vi "TSCAN_GetCANDBInfo.vi"(8 "ADatabaseld":u32=1, 10 "Path":path) -> (0 "ID":i32[](array[numeric]) format="%x", 1 "SignalName":string[][](array[string]), 2 "Message":string[](array[string]), 3 "Path output":path, 4 "Message&ID":string[](array[string]), 5 "ALLName":string[](array[string]))   [LabVIEW 2014]
uses:
  <vilib>/Utility/importsl/GetValueByPointer/GetValueByPointer.xnode
  <vilib>/Utility/importsl/GetValueByPointer/datatype.ctl
panel:
  in  "QueryType":i32(ring) items=["DT_STR_Network_Name", "DT_STR_DBC_FileName", "DT_INT_Protocol_Type", "DT_INT_3", "DT_INT_4", "DT_INT_5", "DT_INT_6", "DT_INT_7", "DT_INT_8", "DT_INT_9", "DT_INT_Signal_List_Count", "DT_INT_CAN_Message_List_Count", "DT_INT_CANFD_Message_List_Count", "DT_INT_CANJ1939_Message_List_Count", "DT_INT_Node_List_Count", "DT_INT_EnvVar_List_Count", "DT_INT_ValTab_List_Count", "DT_INT_17", "DT_INT_18", "DT_INT_19", "DT_INT_Signal_List_Message_ID", "DT_INT_Signal_List_Value_Type", "DT_INT_Signal_List_Is_Motorola", "DT_INT_Signal_List_ValTab_Index", "DT_INT_Signal_List_Mux_Type", "DT_INT_Signal_List_Mux_Value", "DT_INT_Signal_List_Layout_Start", "DT_INT_Signal_List_Length", "DT_DBL_Signal_List_Factor", "DT_DBL_Signal_List_Offset", "DT_DBL_Signal_List_InitValue", "DT_DBL_Signal_List_Min", "DT_DBL_Signal_List_Max", "DT_STR_Signal_List_Name", "DT_STR_Signal_List_Unit", "DT_STR_Signal_List_Comment", "DT_INT_Signal_List_Message_Index", "DT_INT_Signal_List_Message_Type", "DT_STR_Signal_List_Struct", "DT_INT_39", "DT_INT_CAN_Message_List_Type", "DT_INT_CAN_Message_List_DLC", "DT_INT_CAN_Message_List_ID", "DT_INT_CAN_Message_List_CycleTime", "DT_STR_CAN_Message_List_Name", "DT_STR_CAN_Message_List_Comment", "DT_INT_CAN_Message_List_TX_Node_Index", "DT_INT_CAN_Message_List_Owned_Signal_List_Count", "DT_INT_CAN_Message_List_Owned_Signal_List_Signal_Index", "DT_STR_CAN_Message_List_Struct", "DT_INT_50", "DT_INT_51", "DT_INT_52", "DT_INT_53", "DT_INT_54", "DT_INT_55", "DT_INT_56", "DT_INT_57", "DT_INT_58", "DT_INT_59", "DT_INT_CANFD_Message_List_Type", "DT_INT_CANFD_Message_List_DLC", "DT_INT_CANFD_Message_List_ID", "DT_INT_CANFD_Message_List_CycleTime", "DT_STR_CANFD_Message_List_Name", "DT_STR_CANFD_Message_List_Comment", "DT_INT_CANFD_Message_List_TX_Node_Index", "DT_INT_CANFD_Message_List_Owned_Signal_List_Count", "DT_INT_CANFD_Message_List_Owned_Signal_List_Signal_Index", "DT_INT_CANFD_Message_List_BRS", "DT_STR_CANFD_Message_List_Struct", "DT_INT_71", "DT_INT_72", "DT_INT_73", "DT_INT_74", "DT_INT_75", "DT_INT_76", "DT_INT_77", "DT_INT_78", "DT_INT_79", "DT_INT_J1939_Message_List_Type", "DT_INT_J1939_Message_List_DLC", "DT_INT_J1939_Message_List_ID", "DT_INT_J1939_Message_List_CycleTime", "DT_STR_J1939_Message_List_Name", "DT_STR_J1939_Message_List_Comment", "DT_INT_J1939_Message_List_TX_Node_Index", "DT_INT_J1939_Message_List_Owned_Signal_List_Count", "DT_INT_J1939_Message_List_Owned_Signal_List_Signal_Index", "DT_STR_J1939_Message_List_Struct", "DT_INT_90", "DT_INT_91", "DT_INT_92", "DT_INT_93", "DT_INT_94", "DT_INT_95", "DT_INT_96", "DT_INT_97", "DT_INT_98", "DT_INT_99", "DT_INT_Node_List_Address", "DT_STR_Node_List_Name", "DT_STR_Node_List_Comment", "DT_INT_Node_List_TX_CAN_Message_List_Count", "DT_INT_Node_List_TX_CAN_Message_List_Message_Index", "DT_INT_Node_List_RX_CAN_Message_List_Count", "DT_INT_Node_List_RX_CAN_Message_List_Message_Index", "DT_INT_Node_List_TX_FD_Message_List_Count", "DT_INT_Node_List_TX_FD_Message_List_Message_Index", "DT_INT_Node_List_RX_FD_Message_List_Count", "DT_INT_Node_List_RX_FD_Message_List_Message_Index", "DT_INT_Node_List_TX_J1939_Message_List_Count", "DT_INT_Node_List_TX_J1939_Message_List_Message_Index", "DT_INT_Node_List_RX_J1939_Message_List_Count", "DT_INT_Node_List_RX_J1939_Message_List_Message_Index", "DT_INT_Node_List_TX_Signal_List_Count", "DT_INT_Node_List_TX_Signal_List_Signal_Index", "DT_INT_Node_List_RX_Signal_List_Count", "DT_INT_Node_List_RX_Signal_List_Signal_Index", "DT_STR_Node_List_Struct", "DT_INT_120", "DT_INT_121", "DT_INT_122", "DT_INT_123", "DT_INT_124", "DT_INT_125", "DT_INT_126", "DT_INT_127", "DT_INT_128", "DT_INT_129", "DT_INT_EnvVar_List_Value_Type", "DT_DBL_EnvVar_List_MIN", "DT_DBL_EnvVar_List_MAX", "DT_DBL_EnvVar_List_Init_Value", "DT_STR_EnvVar_List_Name", "DT_STR_EnvVar_List_Unit", "DT_STR_EnvVar_List_Comment", "DT_STR_EnvVar_List_Struct", "DT_INT_138", "DT_INT_139", "DT_INT_ValTab_List_Item_List_Count", "DT_INT_ValTab_List_Item_List_Name", "DT_DBL_ValTab_List_Item_List_Value", "DT_STR_ValTab_List_Struct"]
  out "错误输出":errorcluster
  out "tsdb_load_can_db 2":i32
  out "tsdb_load_can_db":i32
  # "Same Mssage in the same row"
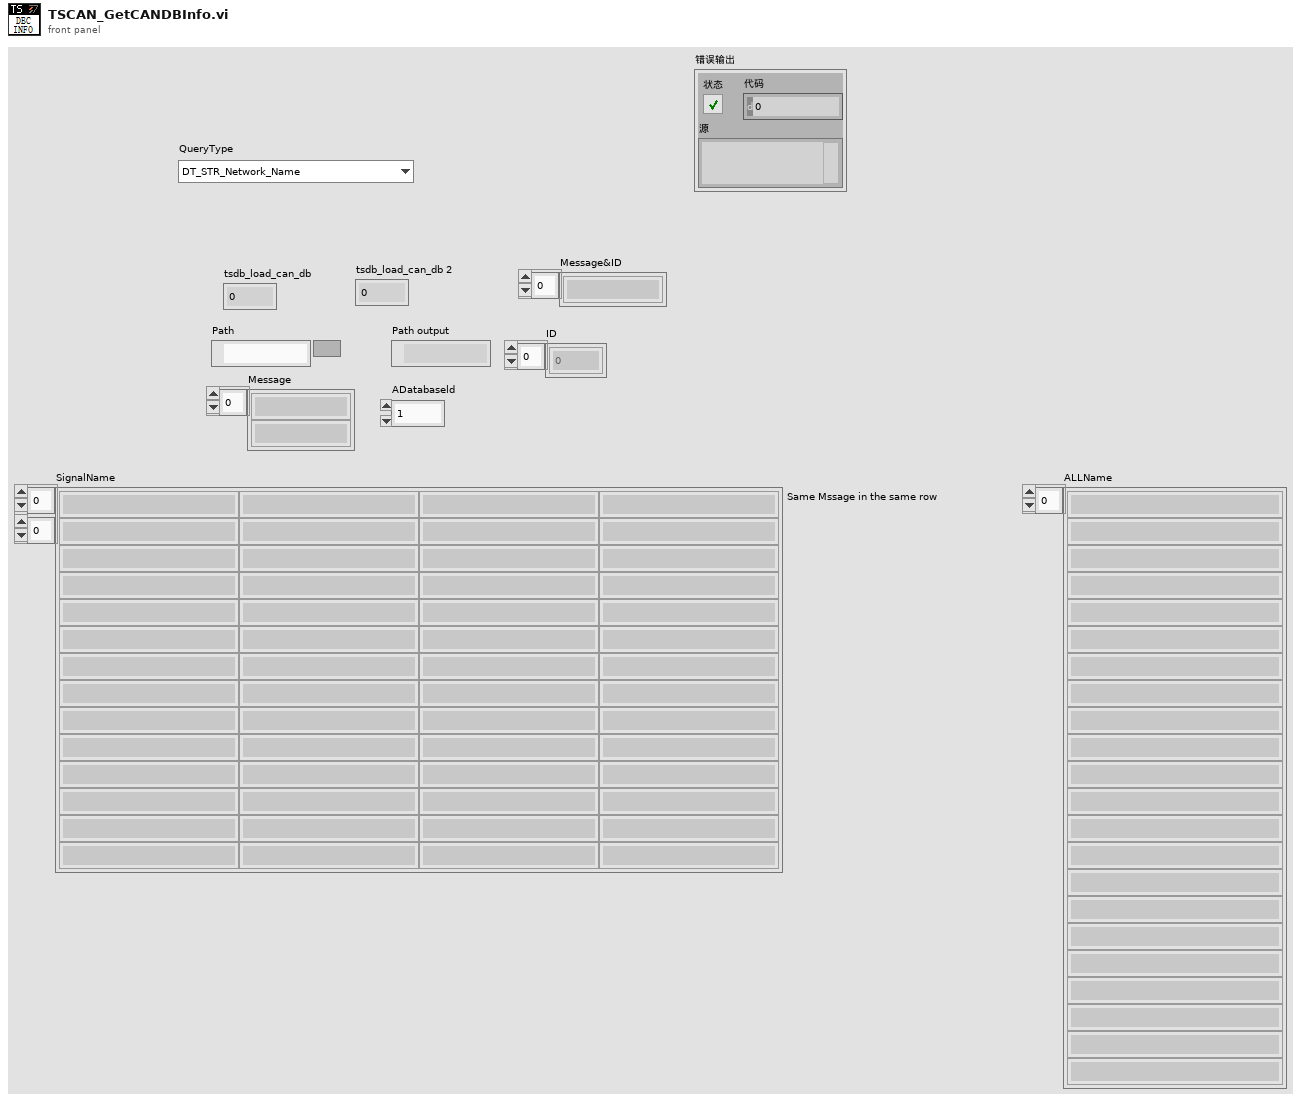
[diagram p1: front panel]
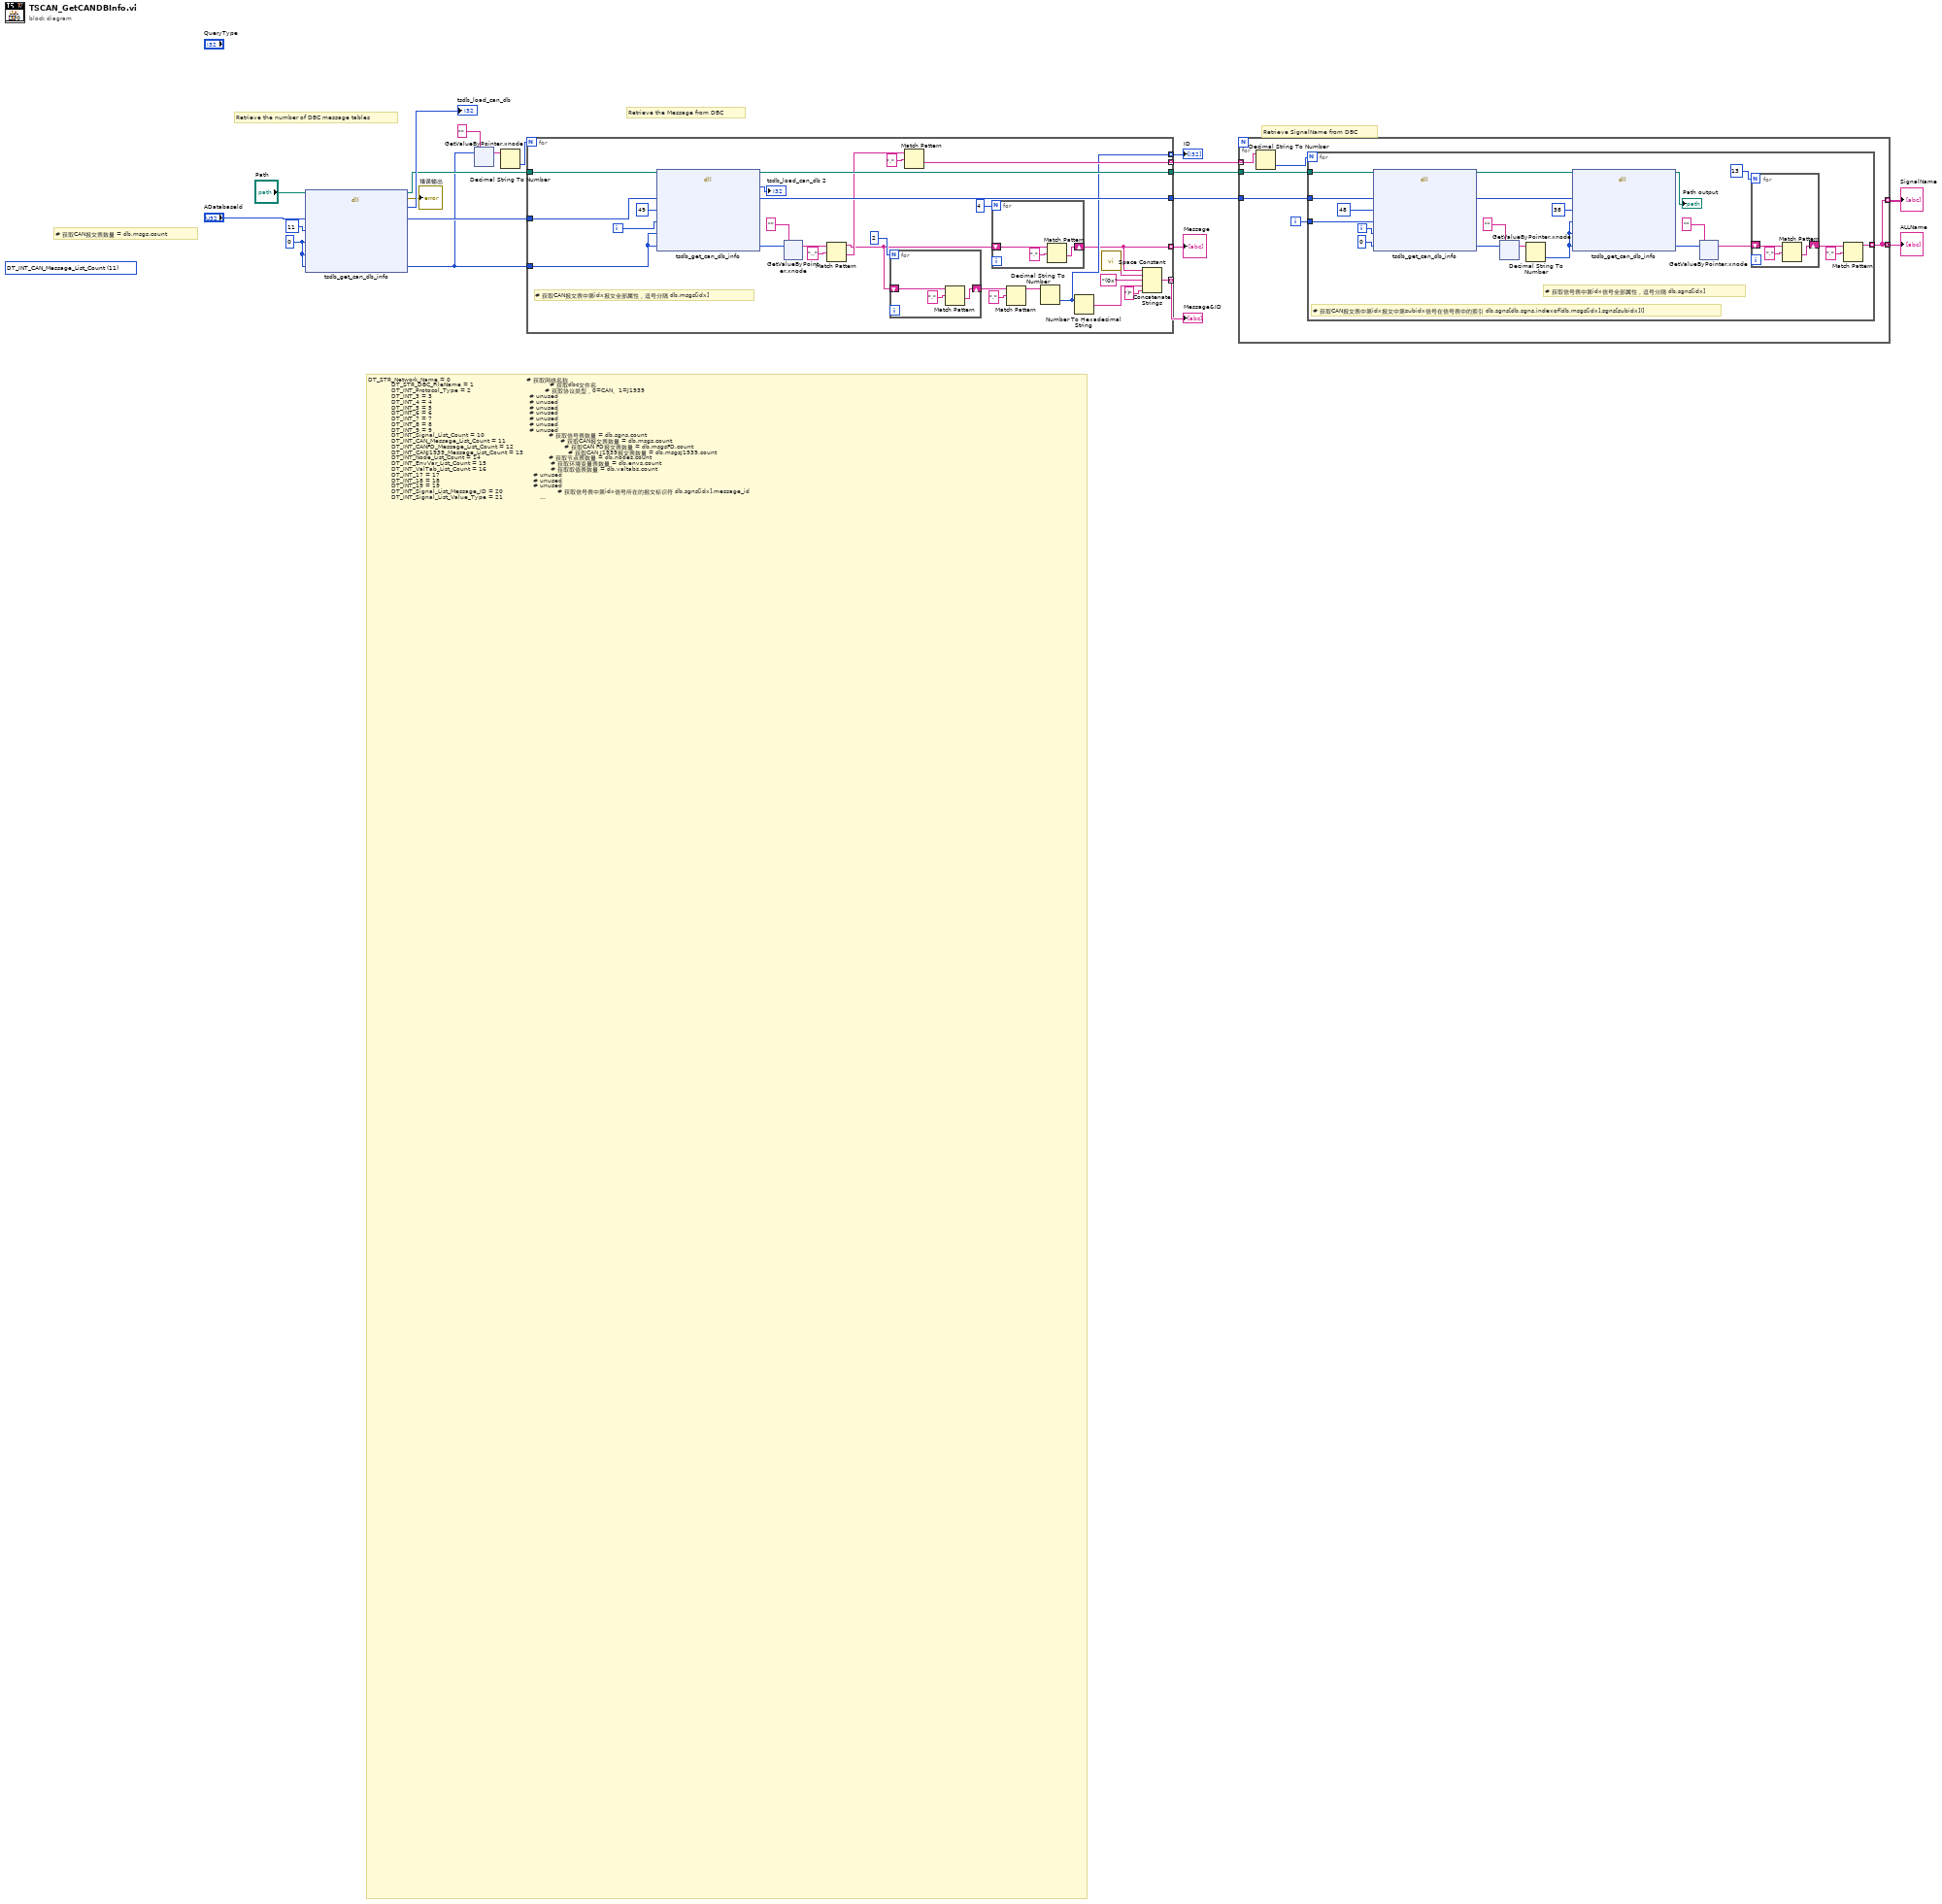
[diagram p0: block diagram]
diagram:
  (unwired) 11 items=["DT_STR_Network_Name", "DT_STR_DBC_FileName", "DT_INT_Protocol_Type", "DT_INT_3", "DT_INT_4", "DT_INT_5", "DT_INT_6", "DT_INT_7", "DT_INT_8", "DT_INT_9", "DT_INT_Signal_List_Count", "DT_INT_CAN_Message_List_Count", "DT_INT_CANFD_Message_List_Count", "DT_INT_CANJ1939_Message_List_Count", "DT_INT_Node_List_Count", "DT_INT_EnvVar_List_Count", "DT_INT_ValTab_List_Count", "DT_INT_17", "DT_INT_18", "DT_INT_19", "DT_INT_Signal_List_Message_ID", "DT_INT_Signal_List_Value_Type", "DT_INT_Signal_List_Is_Motorola", "DT_INT_Signal_List_ValTab_Index", "DT_INT_Signal_List_Mux_Type", "DT_INT_Signal_List_Mux_Value", "DT_INT_Signal_List_Layout_Start", "DT_INT_Signal_List_Length", "DT_DBL_Signal_List_Factor", "DT_DBL_Signal_List_Offset", "DT_DBL_Signal_List_InitValue", "DT_DBL_Signal_List_Min", "DT_DBL_Signal_List_Max", "DT_STR_Signal_List_Name", "DT_STR_Signal_List_Unit", "DT_STR_Signal_List_Comment", "DT_INT_Signal_List_Message_Index", "DT_INT_Signal_List_Message_Type", "DT_STR_Signal_List_Struct", "DT_INT_39", "DT_INT_CAN_Message_List_Type", "DT_INT_CAN_Message_List_DLC", "DT_INT_CAN_Message_List_ID", "DT_INT_CAN_Message_List_CycleTime", "DT_STR_CAN_Message_List_Name", "DT_STR_CAN_Message_List_Comment", "DT_INT_CAN_Message_List_TX_Node_Index", "DT_INT_CAN_Message_List_Owned_Signal_List_Count", "DT_INT_CAN_Message_List_Owned_Signal_List_Signal_Index", "DT_STR_CAN_Message_List_Struct", "DT_INT_50", "DT_INT_51", "DT_INT_52", "DT_INT_53", "DT_INT_54", "DT_INT_55", "DT_INT_56", "DT_INT_57", "DT_INT_58", "DT_INT_59", "DT_INT_CANFD_Message_List_Type", "DT_INT_CANFD_Message_List_DLC", "DT_INT_CANFD_Message_List_ID", "DT_INT_CANFD_Message_List_CycleTime", "DT_STR_CANFD_Message_List_Name", "DT_STR_CANFD_Message_List_Comment", "DT_INT_CANFD_Message_List_TX_Node_Index", "DT_INT_CANFD_Message_List_Owned_Signal_List_Count", "DT_INT_CANFD_Message_List_Owned_Signal_List_Signal_Index", "DT_INT_CANFD_Message_List_BRS", "DT_STR_CANFD_Message_List_Struct", "DT_INT_71", "DT_INT_72", "DT_INT_73", "DT_INT_74", "DT_INT_75", "DT_INT_76", "DT_INT_77", "DT_INT_78", "DT_INT_79", "DT_INT_J1939_Message_List_Type", "DT_INT_J1939_Message_List_DLC", "DT_INT_J1939_Message_List_ID", "DT_INT_J1939_Message_List_CycleTime", "DT_STR_J1939_Message_List_Name", "DT_STR_J1939_Message_List_Comment", "DT_INT_J1939_Message_List_TX_Node_Index", "DT_INT_J1939_Message_List_Owned_Signal_List_Count", "DT_INT_J1939_Message_List_Owned_Signal_List_Signal_Index", "DT_STR_J1939_Message_List_Struct", "DT_INT_90", "DT_INT_91", "DT_INT_92", "DT_INT_93", "DT_INT_94", "DT_INT_95", "DT_INT_96", "DT_INT_97", "DT_INT_98", "DT_INT_99", "DT_INT_Node_List_Address", "DT_STR_Node_List_Name", "DT_STR_Node_List_Comment", "DT_INT_Node_List_TX_CAN_Message_List_Count", "DT_INT_Node_List_TX_CAN_Message_List_Message_Index", "DT_INT_Node_List_RX_CAN_Message_List_Count", "DT_INT_Node_List_RX_CAN_Message_List_Message_Index", "DT_INT_Node_List_TX_FD_Message_List_Count", "DT_INT_Node_List_TX_FD_Message_List_Message_Index", "DT_INT_Node_List_RX_FD_Message_List_Count", "DT_INT_Node_List_RX_FD_Message_List_Message_Index", "DT_INT_Node_List_TX_J1939_Message_List_Count", "DT_INT_Node_List_TX_J1939_Message_List_Message_Index", "DT_INT_Node_List_RX_J1939_Message_List_Count", "DT_INT_Node_List_RX_J1939_Message_List_Message_Index", "DT_INT_Node_List_TX_Signal_List_Count", "DT_INT_Node_List_TX_Signal_List_Signal_Index", "DT_INT_Node_List_RX_Signal_List_Count", "DT_INT_Node_List_RX_Signal_List_Signal_Index", "DT_STR_Node_List_Struct", "DT_INT_120", "DT_INT_121", "DT_INT_122", "DT_INT_123", "DT_INT_124", "DT_INT_125", "DT_INT_126", "DT_INT_127", "DT_INT_128", "DT_INT_129", "DT_INT_EnvVar_List_Value_Type", "DT_DBL_EnvVar_List_MIN", "DT_DBL_EnvVar_List_MAX", "DT_DBL_EnvVar_List_Init_Value", "DT_STR_EnvVar_List_Name", "DT_STR_EnvVar_List_Unit", "DT_STR_EnvVar_List_Comment", "DT_STR_EnvVar_List_Struct", "DT_INT_138", "DT_INT_139", "DT_INT_ValTab_List_Item_List_Count", "DT_INT_ValTab_List_Item_List_Name", "DT_DBL_ValTab_List_Item_List_Value", "DT_STR_ValTab_List_Struct"] ("QueryType")
  w8 = u32 0 ("AIndex")
  # "# 获取CAN报文表数量 = db.msgs.count"
  # "DT_STR_Network_Name = 0                                       # 获取网络名称\n            DT_STR_DBC_FileName = 1                                       # 获取dbc文件名\n            DT_INT_Protocol_Type = 2                                      # 获取协议类型，0=CAN、1=J1939\n            DT_INT_3 = 3                                                  # unused\n            DT_INT_4 = 4                                                  # unused\n            DT_INT_5 = 5                                                  # unused\n            DT_INT_6 = 6                                                  # unused\n            DT_INT_7 = 7                                                  # unused\n            DT_INT_8 = 8                                                  # unused\n            DT_INT_9 = 9                                                  # unused\n            DT_INT_Signal_List_Count = 10                                 # 获取信号表数量 = db.sgns.count\n            DT_INT_CAN_Message_List_Count = 11                            # 获取CAN报文表数量 = db.msgs.count\n            DT_INT_CANFD_Message_List_Count = 12                          # 获取CAN FD报文表数量 = db.msgsFD.count\n            DT_INT_CANJ1939_Message_List_Count = 13                       # 获取CAN J1939报文表数量 = db.msgsJ1939.count\n            DT_INT_Node_List_Count = 14                                   # 获取节点表数量 = db.nodes.count\n            DT_INT_EnvVar_List_Count = 15                                 # 获取环境变量表数量 = db.envs.count\n            DT_INT_ValTab_List_Count = 16                                 # 获取取值表数量 = db.valtabs.count\n            DT_INT_17 = 17                                                # unused\n            DT_INT_18 = 18                                                # unused\n            DT_INT_19 = 19                                                # unused\n            DT_INT_Signal_List_Message_ID = 20                            # 获取信号表中第idx信号所在的报文标识符 db.sgns[idx].message_id\n            DT_INT_Signal_List_Value_Type = 21                            # 获取信号表中第idx信号值类型 0-无符号整型 1-有符号整型 2-32位浮点 3-64位浮点\n            DT_INT_Signal_List_Is_Motorola = 22                           # 获取信号表中第idx信号是否是Motorola格式，0-Intel格式、1-Motorola格式\n            DT_INT_Signal_List_ValTab_Index = 23                          # 获取信号表中第idx信号所带的取值表在取值表列表中的索引\n            DT_INT_Signal_List_Mux_Type = 24                              # 获取信号表中第idx信号Mux类型，0-普通信号 1-multiplexor 2-multiplexed信号\n            DT_INT_Signal_List_Mux_Value = 25                             # 获取信号表中第idx信号作为multiplexor的值\n            DT_INT_Signal_List_Layout_Start = 26                          # 获取信号表中第idx信号在报文中的起始位\n            DT_INT_Signal_List_Length = 27                                # 获取信号表中第idx信号的信号长度\n            DT_DBL_Signal_List_Factor = 28                                # 获取信号表中第idx信号放大因子\n            DT_DBL_Signal_List_Offset = 29                                # 获取信号表中第idx信号偏移量\n            DT_DBL_Signal_List_InitValue = 30                             # 获取信号表中第idx信号初始值\n            DT_DBL_Signal_List_Min = 31                                   # 获取信号表中第idx信号最小值\n            DT_DBL_Signal_List_Max = 32                                   # 获取信号表中第idx信号最大值\n            DT_STR_Signal_List_Name = 33                                  # 获取信号表中第idx信号名称\n            DT_STR_Signal_List_Unit = 34                                  # 获取信号表中第idx信号单位\n            DT_STR_Signal_List_Comment = 35                               # 获取信号表中第idx信号注释\n            DT_INT_Signal_List_Message_Index = 36                         # 获取信号表中第idx信号所在的报文在报文表中的索引 db.msgs[db.sgns[idx].message_idx]\n            DT_INT_Signal_List_Message_Type = 37                          # 获取信号表中第idx信号所在的报文的类型，0=CAN 1=CANFD 2=J1939\n            DT_STR_Signal_List_Struct = 38                                # 获取信号表中第idx信号全部属性，逗号分隔 db.sgns[idx]\n            DT_INT_39 = 39                                                # unused\n            DT_INT_CAN_Message_List_Type = 40                             # 获取CAN报文表中第idx报文类型，cftStdCAN = 0 cftExtCAN = 1 cftJ1939 = 2 cftStdCANFD = 3 cftExtCANFD = 4\n            DT_INT_CAN_Message_List_DLC = 41                              # 获取CAN报文表中第idx报文数据长度\n            DT_INT_CAN_Message_List_ID = 42                               # 获取CAN报文表中第idx报文标识符\n            DT_INT_CAN_Message_List_CycleTime = 43                        # 获取CAN报文表中第idx报文周期\n            DT_STR_CAN_Message_List_Name = 44                             # 获取CAN报文表中第idx报文名称\n            DT_STR_CAN_Message_List_Comment = 45                          # 获取CAN报文表中第idx报文注释\n            DT_INT_CAN_Message_List_TX_Node_Index = 46                    # 获取CAN报文表中第idx报文对应的发送节点的索引\n            DT_INT_CAN_Message_List_Owned_Signal_List_Count = 47          # 获取CAN报文表中第idx报文拥有的信号数量 db.msgs[idx].sgns.count\n            DT_INT_CAN_Message_List_Owned_Signal_List_Signal_Index = 48   # 获取CAN报文表中第idx报文中第subidx信号在信号表中的索引 db.sgns[db.sgns.indexof(db.msgs[idx].sgns[subidx])]\n            DT_STR_CAN_Message_List_Struct = 49                           # 获取CAN报文表中第idx报文全部属性，逗号分隔 db.msgs[idx]\n            DT_INT_50 = 50                                                # unused\n            DT_INT_51 = 51                                                # unused\n            DT_INT_52 = 52                                                # unused\n            DT_INT_53 = 53                                                # unused\n            DT_INT_54 = 54                                                # unused\n            DT_INT_55 = 55                                                # unused\n            DT_INT_56 = 56                                                # unused\n            DT_INT_57 = 57                                                # unused\n            DT_INT_58 = 58                                                # unused\n            DT_INT_59 = 59                                                # unused\n            DT_INT_CANFD_Message_List_Type = 60                           # 获取CANFD报文表中第idx报文类型，cftStdCAN = 0 cftExtCAN = 1 cftJ1939 = 2 cftStdCANFD = 3 cftExtCANFD = 4\n            DT_INT_CANFD_Message_List_DLC = 61                            # 获取CANFD报文表中第idx报文数据长度\n            DT_INT_CANFD_Message_List_ID = 62                             # 获取CANFD报文表中第idx报文标识符\n            DT_INT_CANFD_Message_List_CycleTime = 63                      # 获取CANFD报文表中第idx报文周期\n            DT_STR_CANFD_Message_List_Name = 64                           # 获取CANFD报文表中第idx报文名称\n            DT_STR_CANFD_Message_List_Comment = 65                        # 获取CANFD报文表中第idx报文注释\n            DT_INT_CANFD_Message_List_TX_Node_Index = 66                  # 获取CANFD报文表中第idx报文对应的发送节点的索引\n            DT_INT_CANFD_Message_List_Owned_Signal_List_Count = 67        # 获取CANFD报文表中第idx报文拥有的信号数量 db.msgs[idx].sgns.count\n            DT_INT_CANFD_Message_List_Owned_Signal_List_Signal_Index = 68 # 获取CANFD报文表中第idx报文中第subidx信号在信号表中的索引 db.sgns[db.sgns.indexof(db.msgs[idx].sgns[subidx])]\n            DT_INT_CANFD_Message_List_BRS = 69                            # 获取CANFD报文表中第idx报文BRS，0-No BRS、1-BRS\n            DT_STR_CANFD_Message_List_Struct = 70                         # 获取CANFD报文表中第idx报文全部属性，逗号分隔 db.msgs[idx]\n            DT_INT_71 = 71                                                # unused\n            DT_INT_72 = 72                                                # unused\n            DT_INT_73 = 73                                                # unused\n            DT_INT_74 = 74                                                # unused\n            DT_INT_75 = 75                                                # unused\n            DT_INT_76 = 76                                                # unused\n            DT_INT_77 = 77                                                # unused\n            DT_INT_78 = 78                                                # unused\n            DT_INT_79 = 79                                                # unused\n            DT_INT_J1939_Message_List_Type = 80                           # 获取J1939报文表中第idx报文类型，cftStdCAN = 0 cftExtCAN = 1 cftJ1939 = 2 cftStdCANFD = 3 cftExtCANFD = 4\n            DT_INT_J1939_Message_List_DLC = 81                            # 获取J1939报文表中第idx报文数据长度\n            DT_INT_J1939_Message_List_ID = 82                             # 获取J1939报文表中第idx报文标识符\n            DT_INT_J1939_Message_List_CycleTime = 83                      # 获取J1939报文表中第idx报文周期\n            DT_STR_J1939_Message_List_Name = 84                           # 获取J1939报文表中第idx报文名称\n            DT_STR_J1939_Message_List_Comment = 85                        # 获取J1939报文表中第idx报文注释\n            DT_INT_J1939_Message_List_TX_Node_Index = 86                  # 获取J1939报文表中第idx报文对应的发送节点的索引\n            DT_INT_J1939_Message_List_Owned_Signal_List_Count = 87        # 获取J1939报文表中第idx报文拥有的信号数量 db.msgs[idx].sgns.count\n            DT_INT_J1939_Message_List_Owned_Signal_List_Signal_Index = 88 # 获取J1939报文表中第idx报文中第subidx信号在信号表中的索引 db.sgns[db.sgns.indexof(db.msgs[idx].sgns[subidx])]\n            DT_STR_J1939_Message_List_Struct = 89                         # 获取CAN报文表中第idx报文全部属性，逗号分隔 db.msgs[idx]\n            DT_INT_90 = 90                                                # unused\n            DT_INT_91 = 91                                                # unused\n            DT_INT_92 = 92                                                # unused\n            DT_INT_93 = 93                                                # unused\n            DT_INT_94 = 94                                                # unused\n            DT_INT_95 = 95                                                # unused\n            DT_INT_96 = 96                                                # unused\n            DT_INT_97 = 97                                                # unused\n            DT_INT_98 = 98                                                # unused\n            DT_INT_99 = 99                                                # unused\n            DT_INT_Node_List_Address = 100                                # 获取节点表中第idx节点地址，默认为0\n            DT_STR_Node_List_Name = 101                                   # 获取节点表中第idx节点名称\n            DT_STR_Node_List_Comment = 102                                # 获取节点表中第idx节点注释\n            DT_INT_Node_List_TX_CAN_Message_List_Count = 103              # 获取节点表中第idx节点所发送的CAN报文数量 db.nodes[idx].txmsgs.count\n            DT_INT_Node_List_TX_CAN_Message_List_Message_Index = 104      # 获取节点表中第idx节点所发送的subidx报文在CAN报文表中的索引 db.msgs[db.msgs.indexof(db.nodes[idx].txmsgs[subidx])]\n            DT_INT_Node_List_RX_CAN_Message_List_Count = 105              # 获取节点表中第idx节点所接收的CAN报文数量\n            DT_INT_Node_List_RX_CAN_Message_List_Message_Index = 106      # 获取节点表中第idx节点所接收的subidx报文在CAN报文表中的索引\n            DT_INT_Node_List_TX_FD_Message_List_Count = 107               # 获取节点表中第idx节点所发送的FD报文数量 db.nodes[idx].txmsgs.count\n            DT_INT_Node_List_TX_FD_Message_List_Message_Index = 108       # 获取节点表中第idx节点所发送的subidx报文在FD报文表中的索引 db.msgs[db.msgs.indexof(db.nodes[idx].txmsgs[subidx])]\n            DT_INT_Node_List_RX_FD_Message_List_Count = 109               # 获取节点表中第idx节点所接收的FD报文数量\n            DT_INT_Node_List_RX_FD_Message_List_Message_Index = 110       # 获取节点表中第idx节点所接收的subidx报文在FD报文表中的索引\n            DT_INT_Node_List_TX_J1939_Message_List_Count = 111            # 获取节点表中第idx节点所发送的J1939报文数量 db.nodes[idx].txmsgs.count\n            DT_INT_Node_List_TX_J1939_Message_List_Message_Index = 112    # 获取节点表中第idx节点所发送的subidx报文在J1939报文表中的索引 db.msgs[db.msgs.indexof(db.nodes[idx].txmsgs[subidx])]\n            DT_INT_Node_List_RX_J1939_Message_List_Count = 113            # 获取节点表中第idx节点所接收的J1939报文数量\n            DT_INT_Node_List_RX_J1939_Message_List_Message_Index = 114    # 获取节点表中第idx节点所接收的subidx报文在J1939报文表中的索引\n            DT_INT_Node_List_TX_Signal_List_Count = 115                   # 获取节点表中第idx节点所发送的信号数量\n            DT_INT_Node_List_TX_Signal_List_Signal_Index = 116            # 获取节点表中第idx节点所发送的subidx信号在信号表中的索引\n            DT_INT_Node_List_RX_Signal_List_Count = 117                   # 获取节点表中第idx节点所接收的信号数量\n            DT_INT_Node_List_RX_Signal_List_Signal_Index = 118            # 获取节点表中第idx节点所接收的subidx信号在信号表中的索引\n            DT_STR_Node_List_Struct = 119                                 # 获取节点表中第idx节点全部属性，逗号分隔 db.nodes[idx]\n            DT_INT_120 = 120                                              # unused\n            DT_INT_121 = 121                                              # unused\n            DT_INT_122 = 122                                              # unused\n            DT_INT_123 = 123                                              # unused\n            DT_INT_124 = 124                                              # unused\n            DT_INT_125 = 125                                              # unused\n            DT_INT_126 = 126                                              # unused\n            DT_INT_127 = 127                                              # unused\n            DT_INT_128 = 128                                              # unused\n            DT_INT_129 = 129                                              # unused\n            DT_INT_EnvVar_List_Value_Type = 130                           # 获取环境变量表中第idx环境变量值类型，0-整型、1-浮点、2-字符串、3-数据\n            DT_DBL_EnvVar_List_MIN = 131                                  # 获取环境变量表中第idx环境变量最小值\n            DT_DBL_EnvVar_List_MAX = 132                                  # 获取环境变量表中第idx环境变量最大值\n            DT_DBL_EnvVar_List_Init_Value = 133                           # 获取环境变量表中第idx环境变量初始值\n            DT_STR_EnvVar_List_Name = 134                                 # 获取环境变量表中第idx环境变量名称\n            DT_STR_EnvVar_List_Unit = 135                                 # 获取环境变量表中第idx环境变量单位\n            DT_STR_EnvVar_List_Comment = 136                              # 获取环境变量表中第idx环境变量注释\n            DT_STR_EnvVar_List_Struct = 137                               # 获取环境变量表中第idx环境变量全部属性，逗号分隔 db.EnvVars[idx]\n            DT_INT_138 = 138                                              # unused\n            DT_INT_139 = 139                                              # unused\n            DT_INT_ValTab_List_Item_List_Count = 140                      # 获取取值表中第idx取值表所包含的值数量\n            DT_INT_ValTab_List_Item_List_Name = 141                       # 获取取值表中第idx取值表名称\n            DT_DBL_ValTab_List_Item_List_Value = 142                      # 获取取值表中第idx取值表中第subidx的值\n            DT_STR_ValTab_List_Struct = 143                               # 获取取值表中第idx取值表全部属性，逗号分隔 db.ValTabs[idx]"
  # "Retrieve SignalName from DBC"
  # "Retrieve the Message from DBC"
  # "Retrieve the number of DBC message tables"
  n1 = dll-call lib="PTH27abs EDemo同星\nTSCAN_V1.0ConfigTSMaster.dll" fn="tsdb_get_can_db_info"(path in="Path", "ADatabaseld"="ADatabaseld", "AType"=u32 11, "AIndex"=w8, "ASubIndex"=w8, "Return"=w8) -> (path out=w15:path, error out=→"错误输出":errorcluster, "tsdb_load_can_db"=→"tsdb_load_can_db":i32, "ADatabaseld"=w16:u32, "Return"=w14:i32)  [unwired: 5 in]
  n2 = xnode "GetValueByPointer.xnode"("Pointer"=w14, "InputType"="" ("参数6")) -> ("Output"=w13:string)  [unwired: 2 in, 1 out]
  n3 = Decimal String To Number(string=w13) -> (number=w12:i32)  [unwired: 2 in, 1 out]
  n4 = for {
    N: w12 -> [_]
    tunnel: w16 -> [w45]
    tunnel: w15 -> [w44]
    tunnel: w14 -> [w39]
    tunnel: [w22] -> w7 mode=indexing
    tunnel: [w29] -> w11 mode=indexing
    tunnel: [w36] -> w10
    tunnel: [w35] -> w9
    tunnel: [w26] -> w4 mode=indexing
    tunnel: [w24] -> w3 mode=indexing
    i -> [w38]
    # "# 获取CAN报文表中第idx报文全部属性，逗号分隔 db.msgs[idx]"
    n5 = dll-call lib="PTH27abs EDemo同星\nTSCAN_V1.0ConfigTSMaster.dll" fn="tsdb_get_can_db_info"(path in=w44, "ADatabaseld"=w45, "AType"=u32 49, "AIndex"=w38, "ASubIndex"=w39, "Return"=w39) -> (path out=w36:path, "tsdb_load_can_db"=→"tsdb_load_can_db 2":i32, "ADatabaseld"=w35:u32, "Return"=w47:i32)  [unwired: 5 in, 1 out]
    n6 = xnode "GetValueByPointer.xnode"("Pointer"=w47, "InputType"="" ("参数6")) -> ("Output"=w41:string)  [unwired: 2 in, 1 out]
    n7 = Match Pattern(string=w41, regular expression=",," ("正则表达式")) -> (before substring=w32:string, after substring=w33:string)  [unwired: 1 in, 2 out]
    n8 = for {
      N: 2 -> [_]
      shift-right: [w49] -> w30
      shift-left: w32 -> [w51]
      n9 = Match Pattern(string=w51, regular expression="," ("正则表达式")) -> (after substring=w49:string)  [unwired: 1 in, 3 out]
    }
    n10 = Match Pattern(string=w33, regular expression="," ("正则表达式")) -> (after substring=w29:string)  [unwired: 1 in, 3 out]
    n11 = for {
      N: 4 -> [_]
      shift-right: [w52] -> w22
      shift-left: w32 -> [w54]
      n12 = Match Pattern(string=w54, regular expression="," ("正则表达式")) -> (after substring=w52:string)  [unwired: 1 in, 3 out]
    }
    n13 = Match Pattern(string=w30, regular expression="," ("正则表达式")) -> (before substring=w27:string)  [unwired: 1 in, 3 out]
    n14 = Decimal String To Number(string=w27) -> (number=w26:i32)  [unwired: 2 in, 1 out]
    n15 = Number To Hexadecimal String(2:w26) -> (0:w25:string)  [unwired: 1 in]
    n16 = call <vilib>:"Space Constant.vi"() -> ("String"=w21:string)
    n17 = Concatenate Strings(w22, w21, "(0x" ("字符串"), w25, ")" ("字符串")) -> (w24:string)
  }
  "Message" <- w7
  "ID" <- w4
  "Message&ID" <- w3
  n18 = for {
    tunnel: w11 -> [w70] mode=indexing
    tunnel: w10 -> [w72]
    tunnel: w9 -> [w71]
    tunnel: [w67] -> w5 mode=indexing
    tunnel: [w67] -> w2 mode=concatenating
    i -> [w68]
    n19 = Decimal String To Number(string=w70) -> (number=w69:i32)  [unwired: 2 in, 1 out]
    n20 = for {
      N: w69 -> [_]
      tunnel: w72 -> [w93]
      tunnel: w71 -> [w92]
      tunnel: [w85] -> w67 mode=indexing
      tunnel: w68 -> [w82]
      i -> [w83]
      # "# 获取信号表中第idx信号全部属性，逗号分隔 db.sgns[idx]"
      # "# 获取CAN报文表中第idx报文中第subidx信号在信号表中的索引 db.sgns[db.sgns.indexof(db.msgs[idx].sgns[subidx])]"
      n21 = dll-call lib="PTH27abs EDemo同星\nTSCAN_V1.0ConfigTSMaster.dll" fn="tsdb_get_can_db_info"(path in=w93, "ADatabaseld"=w92, "AType"=u32 48, "AIndex"=w82, "ASubIndex"=w83, "Return"=u32 0 ("ASubIndex")) -> (path out=w80:path, "ADatabaseld"=w79:u32, "Return"=w89:i32)  [unwired: 6 in, 1 out]
      n22 = xnode "GetValueByPointer.xnode"("Pointer"=w89, "InputType"="" ("参数6")) -> ("Output"=w81:string)  [unwired: 2 in, 1 out]
      n23 = Decimal String To Number(string=w81) -> (number=w77:i32)  [unwired: 2 in, 1 out]
      n24 = dll-call lib="PTH27abs EDemo同星\nTSCAN_V1.0ConfigTSMaster.dll" fn="tsdb_get_can_db_info"(path in=w80, "ADatabaseld"=w79, "AType"=u32 38, "AIndex"=w77, "ASubIndex"=w77, "Return"=w77) -> (path out=→"Path output":path, "Return"=w74:i32)  [unwired: 7 in, 1 out]
      n25 = xnode "GetValueByPointer.xnode"("Pointer"=w74, "InputType"="" ("参数6")) -> ("Output"=w73:string)  [unwired: 2 in, 1 out]
      n26 = for {
        N: 13 -> [_]
        shift-right: [w106] -> w87
        shift-left: w73 -> [w108]
        n27 = Match Pattern(string=w108, regular expression="," ("正则表达式")) -> (after substring=w106:string)  [unwired: 1 in, 3 out]
      }
      n28 = Match Pattern(string=w87, regular expression="," ("正则表达式")) -> (before substring=w85:string)  [unwired: 1 in, 3 out]
    }
  }
  "SignalName" <- w5
  "ALLName" <- w2
